vi "Hexa String To U32 Color.vi"(10 "8 Char Hexa String":string) -> (2 "U32 Color":u32(colorbox))   [LabVIEW 2021, in "Appearance Actor.lvlib" / "Generic Theme.lvclass"]
uses:
  Generic Theme.lvclass
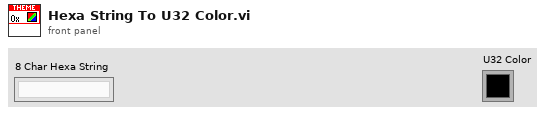
[diagram p1: front panel]
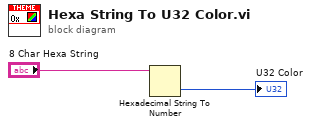
[diagram p0: block diagram]
diagram:
  n1 = Hexadecimal String To Number(string="8 Char Hexa String") -> (number=→"U32 Color":u32)  [unwired: 2 in, 1 out]
